vi "Fetch Data.vi"(7 "Timeout (s)":i32=5, 8 "error out":errorcluster, 10 "Samples":u32=4294967295, 11 "FPGA Session":T1) -> (0 "error out":errorcluster, 2 "Data":u32[](array[numeric]), 3 "FPGA VI Reference Out":T1, 4 "Elements Remaining":u32)   [LabVIEW 2011, in "FlexRIO Host Library (User).lvlib"]
doc: "This VI fetches required number of samples"
uses:
  FlexRIO Host Library (User).lvlib
  <vilib>/rvi/interface/nirviMethod/nirviMethod.xnode
  OCT Reference Design/FPGA Bitfiles/OCTDigitizer_FPGABoard_AcquireDatawitho_CC2D8059.lvbitx
  OCT Reference Design/Complete FPGA Engine/Acquire Data without DRAM.vi
  Session/FPGA Session Ref.ctl
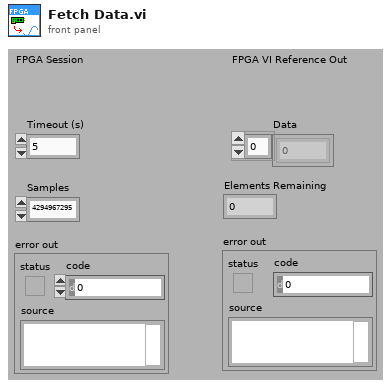
[diagram p1: front panel]
types:
  T1 = typedef "FlexRIO Host Library (User).lvlib/FPGA Session Ref.ctl" = refnum<k20>
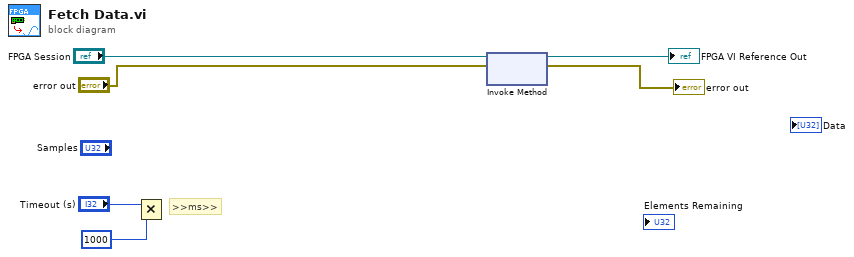
[diagram p0: block diagram]
diagram:
  # ">>ms>>"
  n1 = Multiply(x="Timeout (s)", y=1000) -> (x*y=w6:i32)
  n2 = xnode "Invoke Method"("FPGA VI Reference In"="FPGA Session", "error in"="error out") -> ("FPGA VI Reference Out"=→"FPGA VI Reference Out":T1, "error out"=→"error out":errorcluster)
